vi "PacketHeader.vi"() -> (2 "PacketHeader":string)   [LabVIEW 2017]
uses:
  Typedefs/HW config states enum.ctl
  Global Variables/General Globals.vi
panel:
  out "Found":bool
  out "Expected Control system MAC address":string
  out "Available MAC Addresses":string[](array[string])
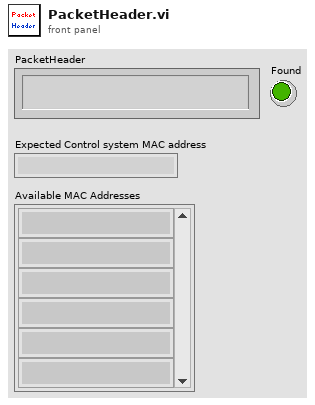
[diagram p1: front panel]
types:
  T1 = typedef "HW config states enum.ctl" = enum16{"Load from file", "Save to file", "Write all", "Read all", "Write XY stage settings", "Write DAQ FPGA settings", "Write Control FPGA settings", "Write Phys Channels", "Write System Config", "Write HW Config", "Save System Config", "Save HW Config", "Clear", "Compare from file"}
  T2 = typedef "Hardware Configuration settings.ctl" = cluster{"Dev. PC":bool, "Swap XY on stage":bool, "No of AOD":u8, "MC Supported":bool, "Axial MC":bool, "Computer MAC address":string, "Externalise Triggers":bool, "Trigger HW config":T3, "DAQmx Chan":T4, "XY stage available":bool, "XY Stage":T5, "Z stage available":bool, "Z Stage config cluster":T6, "Encoder available":bool, "Encoder":T7, "VidRec available":bool, "Cam VidRec":T8, "Laser Power Control HW config":T9, "Laser 1 available":bool, "Laser 1 config cluster":T10, "Prechirper 1 available":bool, "Prechirper 1 config cluster":T11, "Control system.FPGA available?":bool, "Control Sys. HW config":T12, "DAQ FPGA HW Config":T13}
  T3 = typedef "Triggers HW config.ctl" = cluster{"Available Device List":i32, "Device Address":string}
  T4 = typedef "DAQmx physical channels cluster.ctl" = cluster{"Pockels AO":tag, "Hard shutter AO":tag, "PMT AOs":tag, "Galvo AOs":tag, "Power meter AI":tag}
  T5 = typedef "XY Stage config cluster.ctl" = cluster{"COM port":refnum<visa-resource-name>, "Baudrate":i32, "Type":string}
  T6 = typedef "Z Stage config cluster.ctl" = cluster{"COM port":refnum<visa-resource-name>, "Baudrate":i32, "Type":string}
  T7 = typedef "Encoder config cluster.ctl" = cluster{"IP address":string, "Port":u16, "Wheel radius (cm)":dbl, "Encoder Trigger":tag}
  T8 = typedef "Cam VidRec HW config setup cluster.ctl" = cluster{"DO flag-Video record":tag, "DO flag-Trial start":tag}
  T9 = typedef "Laser Power Control HW config.ctl" = cluster{"Laser Power Control":string, "Laser Power Modulation Control":enum16{"NI", "FPGA"}}
  T10 = typedef "Laser 1 config cluster.ctl" = cluster{"COM port":refnum<visa-resource-name>, "Baud Rate":i32, "Type":string}
  T11 = typedef "PreChirper 1 config cluster.ctl" = cluster{"Type":string, "Baud Rate":i32, "COM port":refnum<visa-resource-name>}
  T12 = typedef "Control Sys HW config cluster.ctl" = cluster{"Control system.FPGA Type":enum16{"Virtex 5", "Virtex 7"}, "Control system.Network adapter name":string, "Control system.MAC address":string, "Control system.Ethernet Port":u32, "Control system.Ethernet Port Opened":bool}
  T13 = typedef "DAQ FPGA HW config cluster.ctl" = cluster{"FGPA Ref":T14, "Target":T15, "input card type":T16}
  T14 = typedef "FPGA Ref.ctl" = refnum<k20>
  T15 = typedef "nirio_resource_hc.ctl" = tag
  T16 = typedef "FPGA input type AC-DC.ctl" = enum16{"AC Card", "DC Card"}
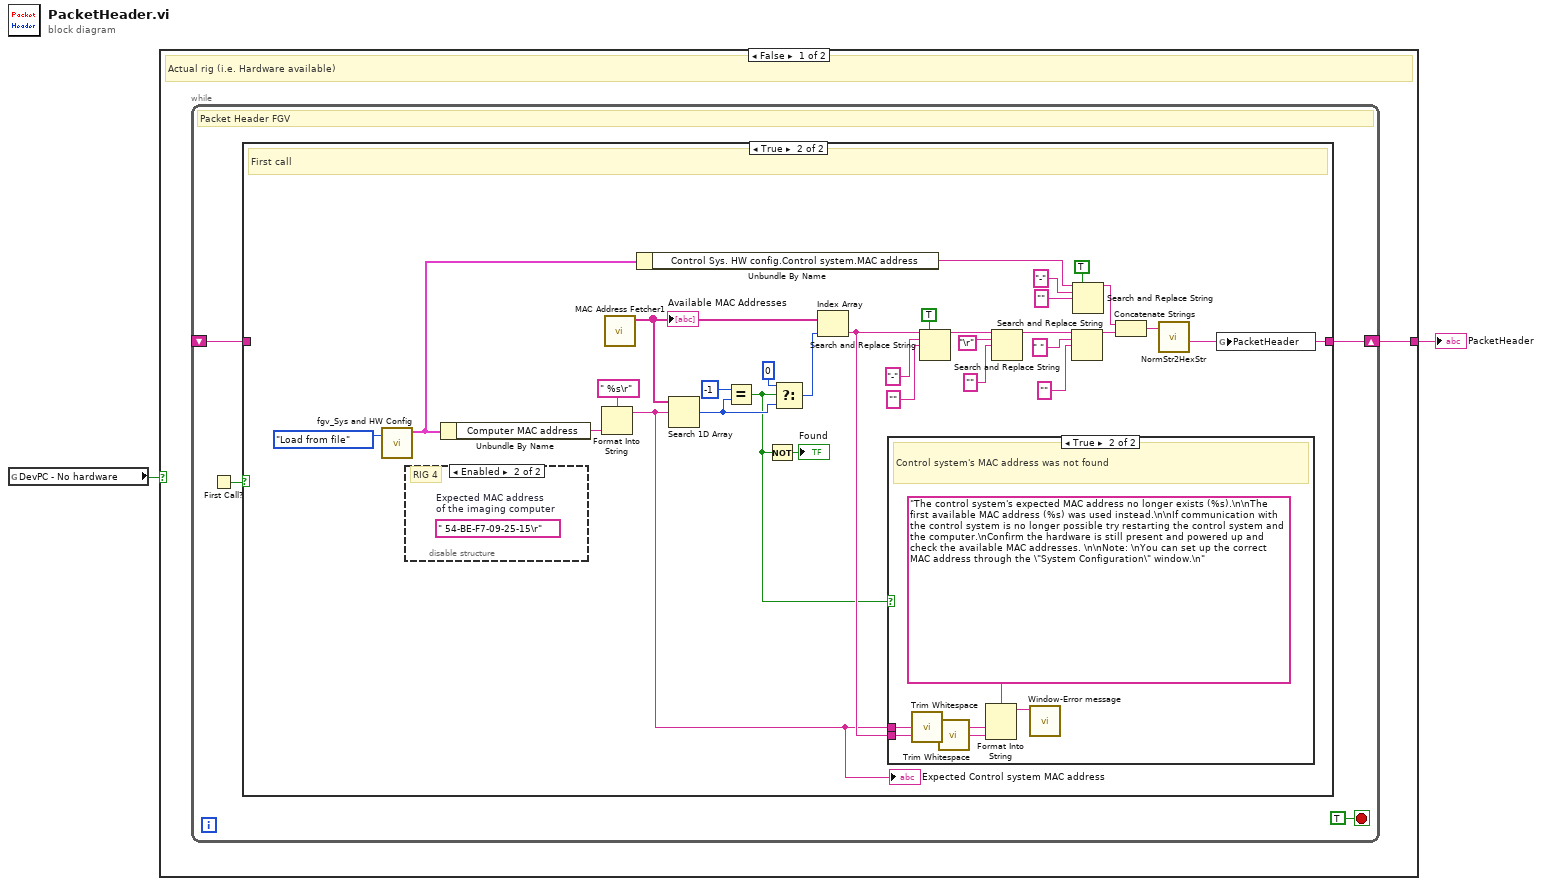
[diagram p0: block diagram]
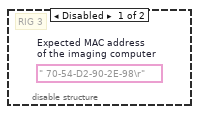
[diagram p3: hidden frame]
diagram:
  n1 = global read "General Globals.vi" "DevPC - No hardware"() -> (w1:bool)
  n2 = case shown="False" w1 {
    tunnel: [w3 _] -> w2
    frame False {
      # "Actual rig (i.e. Hardware available)"
      n3 = while {
        shift-right: [w6] -> w3
        shift-left: _ -> [w5]
        stop <- TRUE stop-if-true
        # "Packet Header FGV"
        n4 = First Call?() -> (First Call?: T/F=w4:bool)
        n5 = case shown="True" w4 {
          tunnel: [w8 w16] -> w6
          tunnel: w5 -> [w8 _]
          frame False {
            # "Not the first call"
          }
          frame True {
            # "First call"
            n6 = call "fgv_Sys and HW Config.vi"("Function"=HW_config_states_enum."Load from file") -> ("Hardware Configuration OUT"=w10:T2)  [unwired: 8 in, 2 out]
            n7 = disable-structure shown="Enabled" {
              frame Disabled {
                (unwired) " 70-54-D2-90-2E-98\r"  # Expected MAC address of the imaging computer
                # "RIG 3"
              }
              frame Enabled {
                (unwired) " 54-BE-F7-09-25-15\r"  # Expected MAC address of the imaging computer
                # "RIG 4"
              }
            }
            n8 = Unbundle By Name(w10) -> ("Computer MAC address"=w9:string)
            n9 = Format Into String(format string=" %s\r" ("Expected MAC address\nof the imaging computer"), w9) -> (resulting string=w13:string)  [unwired: 2 in, 1 out]
            "Expected Control system MAC address" <- w13
            n10 = call "MAC Address Fetcher1.vi"() -> ("MAC Addresses"=w38:string[])  [unwired: 9 in, 2 out]
            "Available MAC Addresses" <- w38
            n11 = Unbundle By Name(w10) -> ("Control Sys. HW config.Control system.MAC address"=w37:string)
            n12 = Search 1D Array(1D array=w38, element=w13) -> (index of element=w19:i32)  [unwired: 1 in]
            n13 = Equal?(x=-1, y=w19) -> (x = y?=w12:bool)
            n14 = Not(x=w12) -> (.not. x?=→"Found":bool)
            n15 = Select(t=0, s=w12, f=w19) -> (s? t:f=w18:i32)
            n16 = Index Array(array=w38, index=w18) -> (element=w17:string)
            n17 = case shown="True" w12 {
              tunnel: w13 -> [_ w42]
              tunnel: w17 -> [_ w41]
              frame False {
                # "Control system's was found"
              }
              frame True {
                # "Control system's MAC address was not found"
                n18 = call <vilib>:"Trim Whitespace.vi"("string"=w42) -> ("trimmed string"=w40:string)  [unwired: 1 in]
                n19 = call <vilib>:"Trim Whitespace.vi"("string"=w41) -> ("trimmed string"=w39:string)  [unwired: 1 in]
                n20 = Format Into String(format string="The control system's expected MAC address no longer exists (%s).\n\nThe first available MAC address (%s) was used instead.\n\nIf communication with the control system is no longer possible try restarting the control system and the computer.\nConfirm the hardware is still present and powered up and check the available MAC addresses. \n\nNote: \nYou can set up the correct MAC address through the \"System Configuration\" window.\n", w40, w39) -> (resulting string=w43:string)  [unwired: 2 in, 1 out]
                n21 = call "Window-Error message.vi"("Message"=w43) -> ()  [unwired: 10 in, 1 out]
              }
            }
            n22 = Search and Replace String(replace all?=TRUE ("replace all? (F)"), input string=w17, search string="-", replace string="" ("replace string (\"\")")) -> (result string=w30:string)  [unwired: 4 in, 3 out]
            n23 = Search and Replace String(input string=w30, search string="\r", replace string="" ("replace string (\"\")")) -> (result string=w24:string)  [unwired: 5 in, 3 out]
            n24 = Search and Replace String(input string=w24, search string=" ", replace string="" ("replace string (\"\")")) -> (result string=w25:string)  [unwired: 5 in, 3 out]
            n25 = Search and Replace String(replace all?=TRUE ("replace all? (F)"), input string=w37, search string="-", replace string="" ("replace string (\"\")")) -> (result string=w27:string)  [unwired: 4 in, 3 out]
            n26 = Concatenate Strings(w27, w25) -> (w26:string)
            n27 = call "NormStr2HexStr.vi"("string"=w26) -> ("hex string"=w16:string)
            n28 = global write "General Globals.vi" "PacketHeader"(w16) -> ()
          }
        }
      }
    }
    frame True {
      # "Development Computer (i.e. No hardware available)"
    }
  }
  "PacketHeader" <- w2
